vi "Write STATUS cluster.vi"(8 "error in (no error)":errorcluster, 10 "STATUS cluster":T1, 11 "PublisherGS in":refnum<class "PublisherGS.lvclass">) -> (0 "error out":errorcluster, 3 "PublisherGS out":refnum<class "PublisherGS.lvclass">)   [LabVIEW 2018, in "PublisherGS.lvclass"]
uses:
  PublisherGS.lvclass
  PublisherGS.lvclass/PublisherGS.ctl
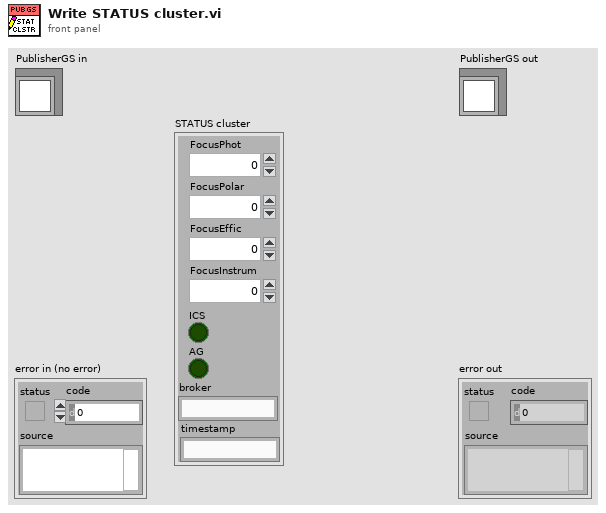
[diagram p1: front panel]
types:
  T1 = cluster{"FocusPhot":dbl, "FocusPolar":dbl, "FocusEffic":dbl, "FocusInstrum":dbl, "ICS":bool, "AG":bool, "broker":string, "timestamp":string}
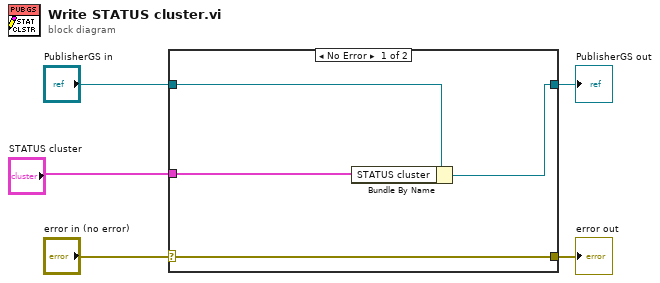
[diagram p0: block diagram]
diagram:
  n1 = case shown="No Error" "error in (no error)" {
    selector: "error in (no error)" -> [w9 w10]
    tunnel: [w9 w10] -> w4
    tunnel: [w7 w11] -> w2
    tunnel: "PublisherGS in" -> [w8 w11]
    tunnel: "STATUS cluster" -> [w6 _]
    frame No Error {
      n2 = Bundle By Name(cluster=w8, "STATUS cluster"=w6) -> (w7:refnum<class "PublisherGS.lvclass">)
    }
    frame Error {
    }
  }
  "error out" <- w4
  "PublisherGS out" <- w2
